vi "Notes Table.vi"(11 "Full Text String Array":string[][](array[string])) -> (0 "Has Annotations?":bool, 1 "Annotation Table":string[][](array[string]), 2 "Times":string[](array[string]), 3 "Labels":string[](array[string]))   [LabVIEW 2021]
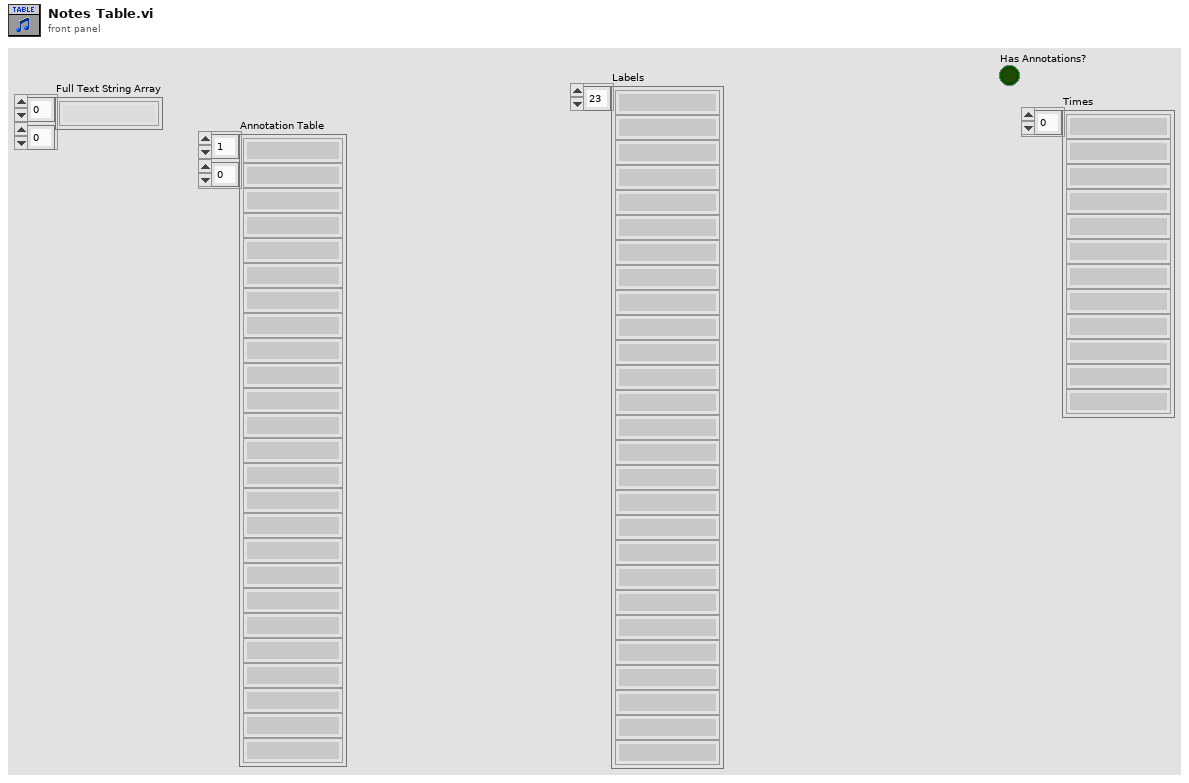
[diagram p1: front panel]
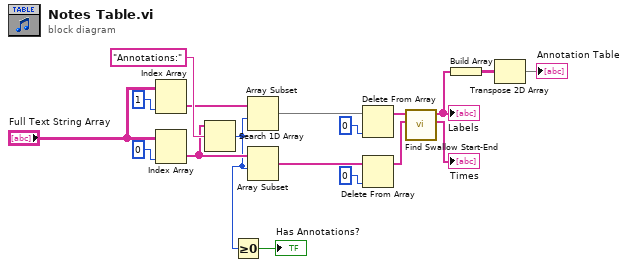
[diagram p0: block diagram]
diagram:
  n1 = Index Array(array="Full Text String Array", index (col)=1 ("disabled index (col)")) -> (element=w12:string[])  [unwired: 1 in]
  n2 = Index Array(array="Full Text String Array", index (col)=0 ("disabled index (col)")) -> (element=w11:string[])  [unwired: 1 in]
  n3 = Search 1D Array(1D array=w11, element="Annotations:") -> (index of element=w2:i32)  [unwired: 1 in]
  n4 = Greater Or Equal To 0?(x=w2) -> (x >= 0?=→"Has Annotations?":bool)
  n5 = Array Subset(array=w12, index=w2) -> (w9:string[])  [unwired: 1 in]
  n6 = Array Subset(array=w11, index=w2) -> (w7:string[])  [unwired: 1 in]
  n7 = Delete From Array(array=w9, index=0) -> (array with subset deleted=w5:string[])  [unwired: 1 in, 1 out]
  n8 = Delete From Array(array=w7, index=0) -> (array with subset deleted=w6:string[])  [unwired: 1 in, 1 out]
  n9 = call "Find Swallow Start-End.vi"("Times"=w6, "Labels"=w5) -> ("Times"=→"Times":string[], "Event Names"=w3:string[])  [unwired: 8 in]
  "Labels" <- w3
  n10 = Build Array(w3) -> (w17:string[][])
  n11 = Transpose 2D Array(2D array=w17) -> (transposed array=→"Annotation Table":string[][])
